vi "NanonisHelper_v1.vi"() -> ()   [LabVIEW 2014]
uses:
  <userlib>/Nanonis Prog Interface V5/Nanonis Prog Interface.lvlib
panel:
  in  "milliseconds to wait":u32=2
  in  "PLL":bool
  in  "size/pixel ratio":bool
  out "TCryo":dbl
  in  "Bias (V)":sgl min=-3.2 max=3.4 format="%#_5p"
  in  "set Bias":bool
  in  "Ratio":enum32{"Equal", "Independent"}(radio)
  out "Path":string="D:\\STM Data\\102016"
  in  "tilt from last image":bool
  out "millisecond timer value":u32=275798
  out "STM [K]":dbl=4.5364351144286035
  in  "polling msec":i32=3000
  in  "Speed (m/s)":cluster{"Forward":sgl, "Backward":sgl}={"Forward"=5.8593752e-08, "Backward"=5.8593752e-08} {"Backward" min=1e-15 max=3.5e-07 format="%.2p"; "Forward" min=1e-15 max=1.5e-07 format="%.2p"}
  in  "Prepare Topos":bool
  in  "Const Height":bool
  out "Saved file path":path=path "D:/STM Data/082016/160804_11-43-53_SPM001.sxm"
  out "Scanning":bool
  in  "up/down":bool=TRUE
  in  "Scan":bool
  in  "STS calc":bool
  in  "Tip cleaner":bool
  out "zdrift m/s":dbl format="%#_5p"
  in  "Duration":dbl
  in  "Z Drift":bool
  in  "stop":bool
  in  "Retract & Center":bool
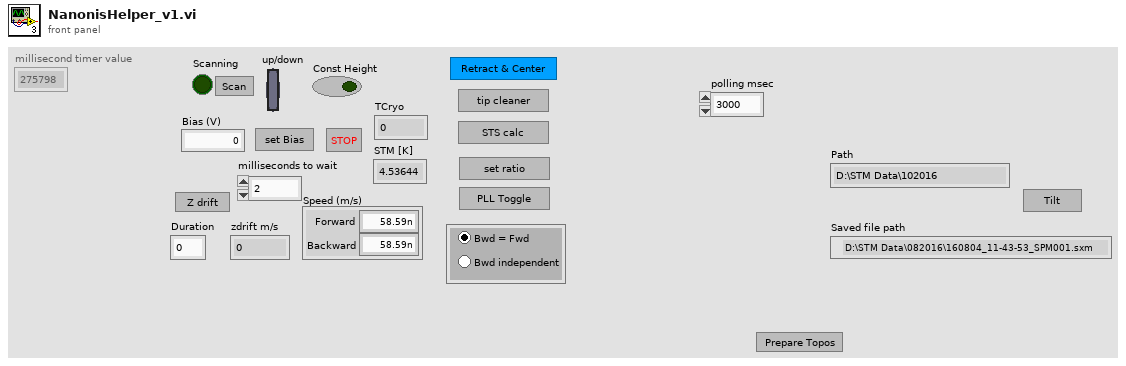
[diagram p1: front panel]
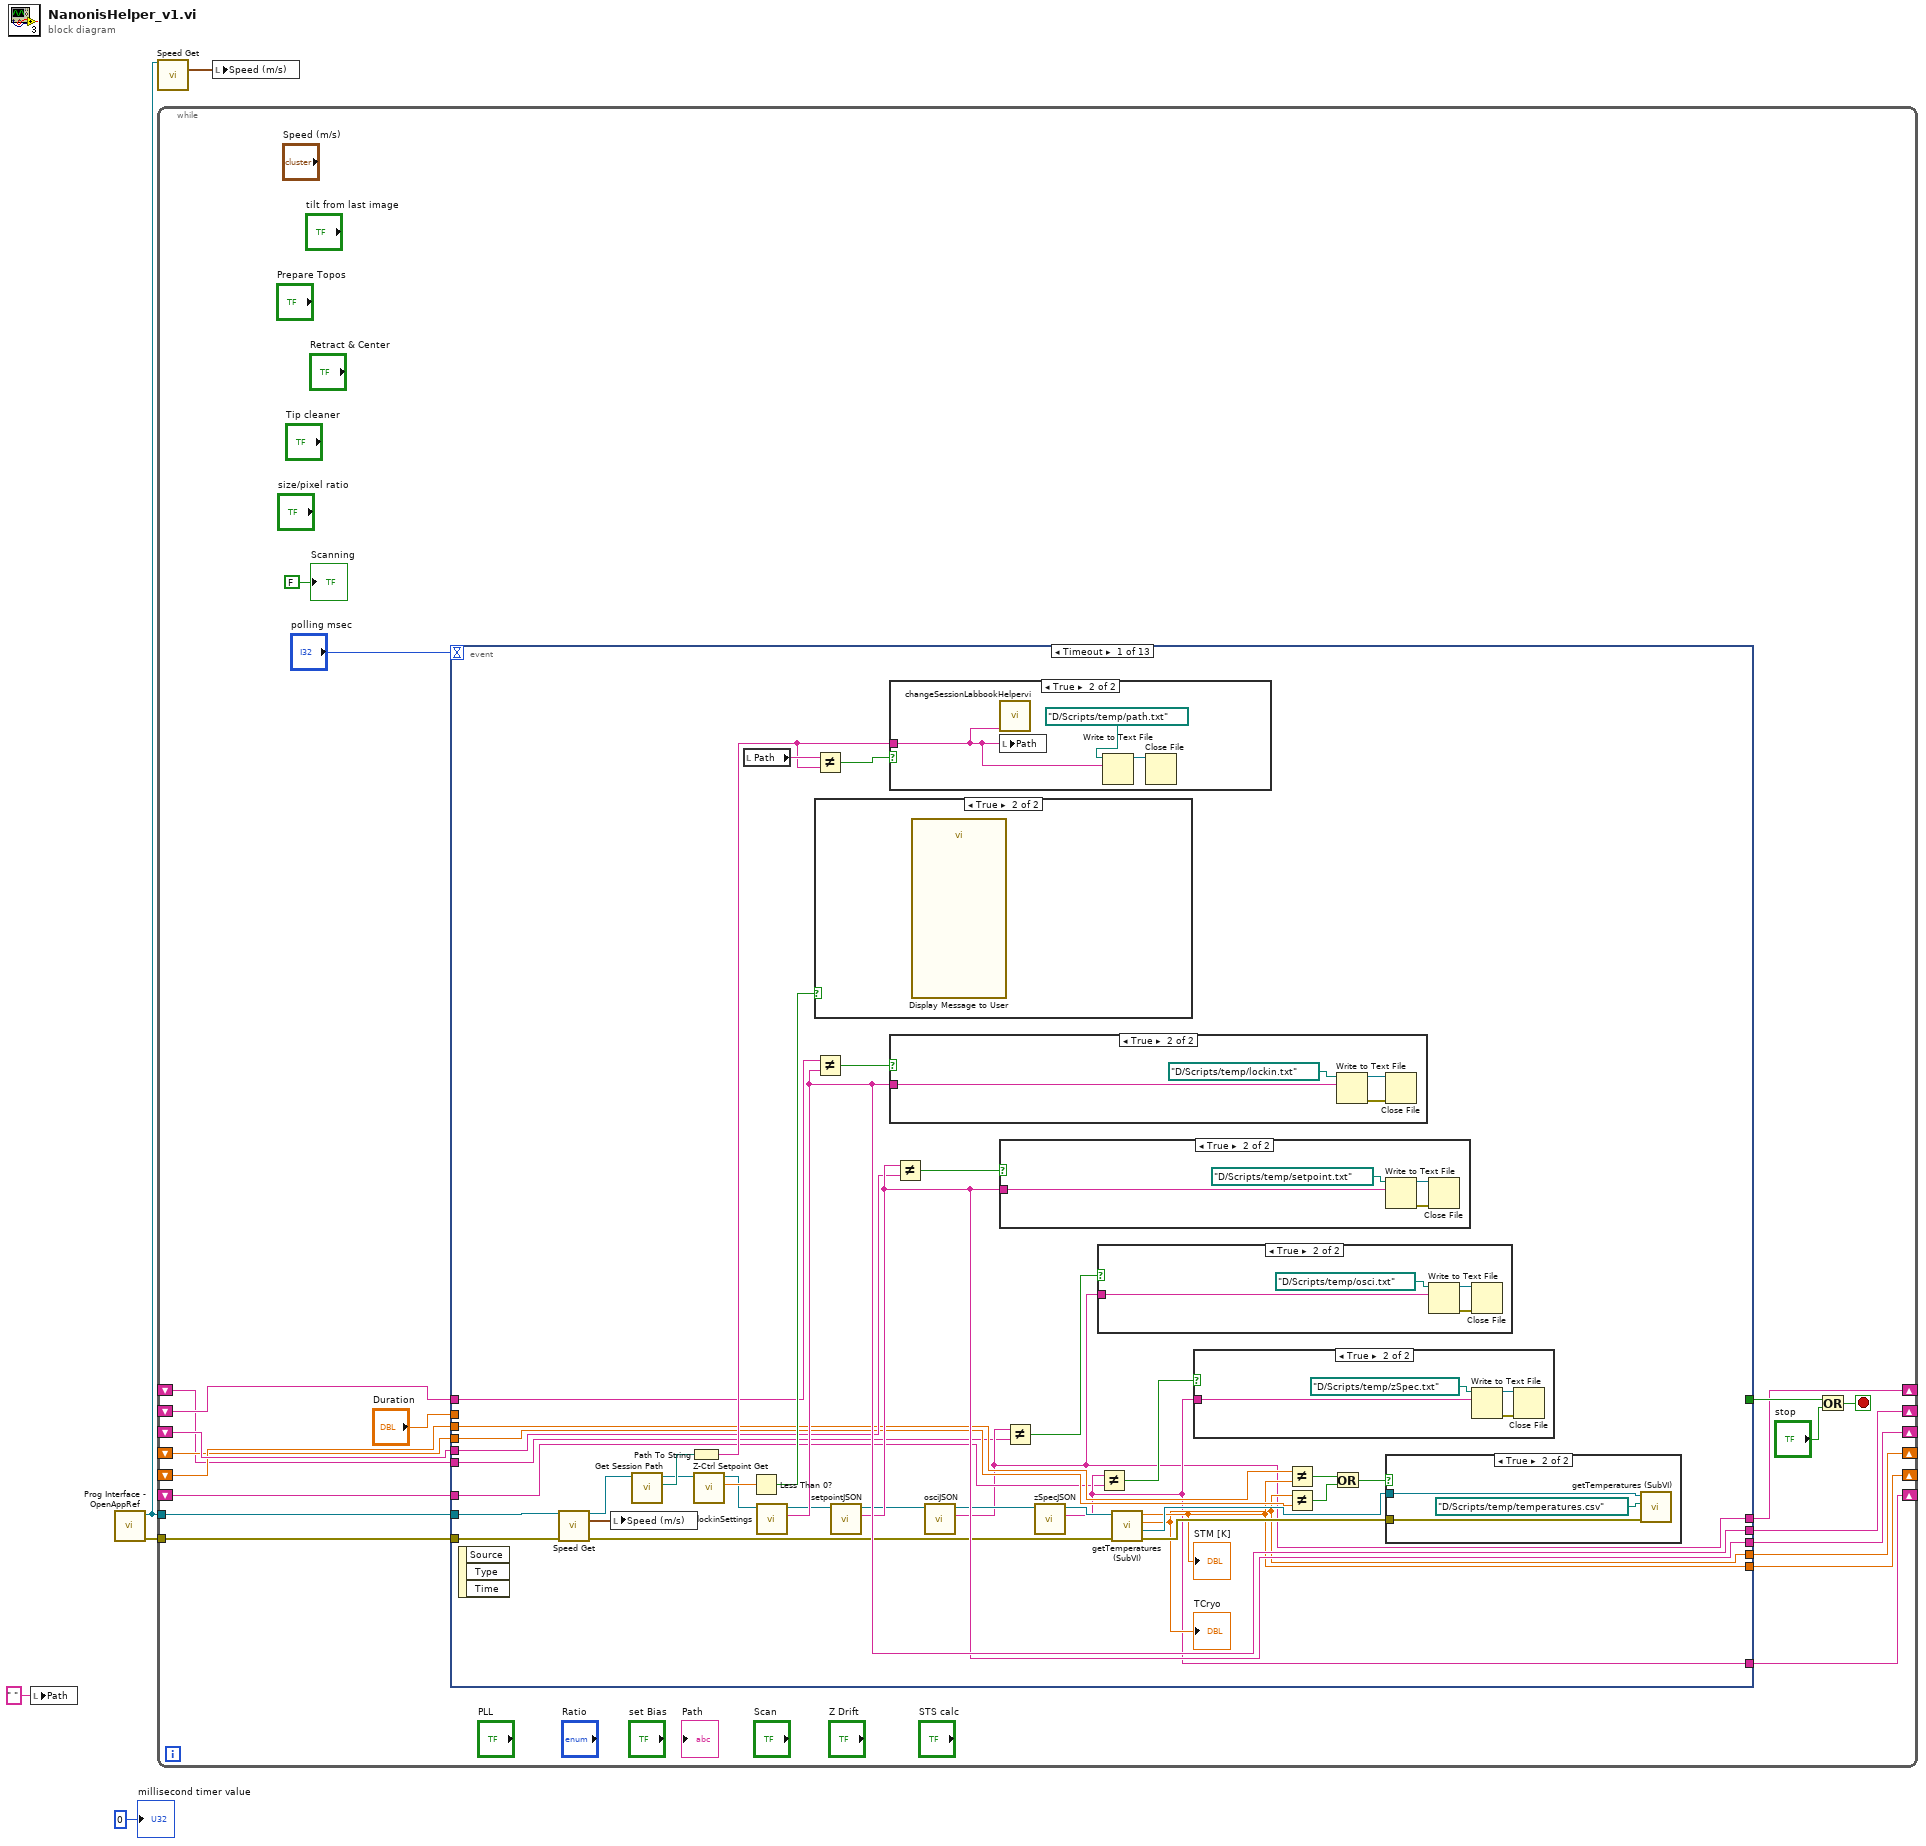
[diagram p0: block diagram]
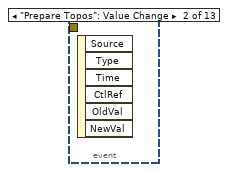
[diagram p9: hidden frame]
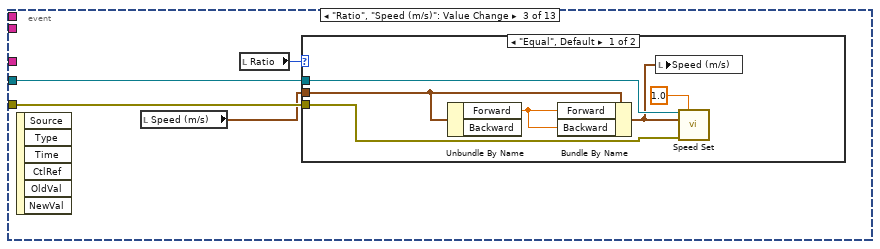
[diagram p10: hidden frame]
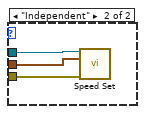
[diagram p11: hidden frame]
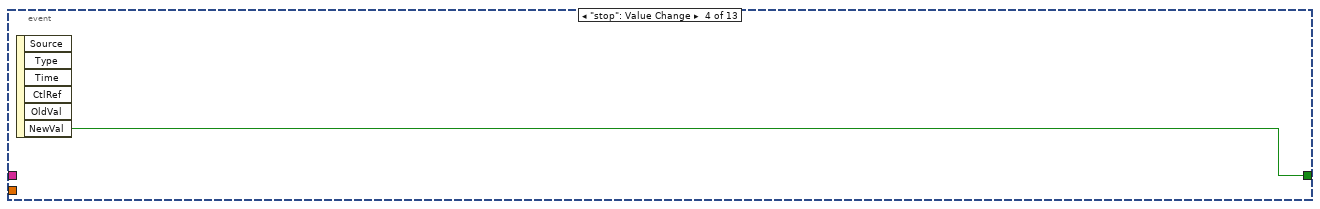
[diagram p12: hidden frame]
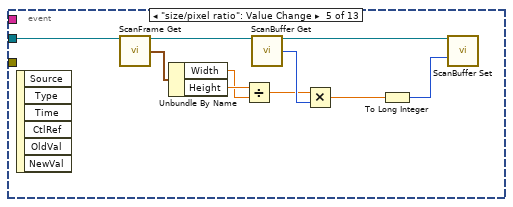
[diagram p13: hidden frame]
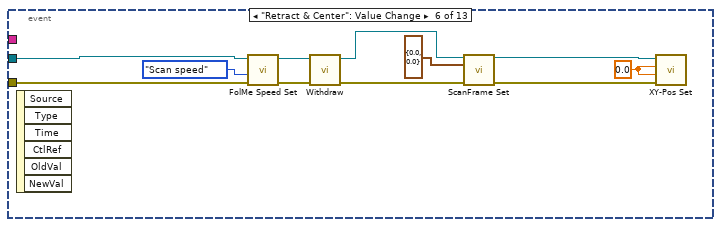
[diagram p14: hidden frame]
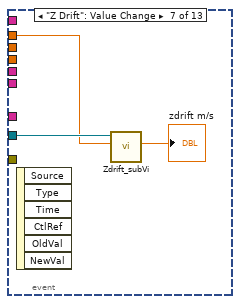
[diagram p15: hidden frame]
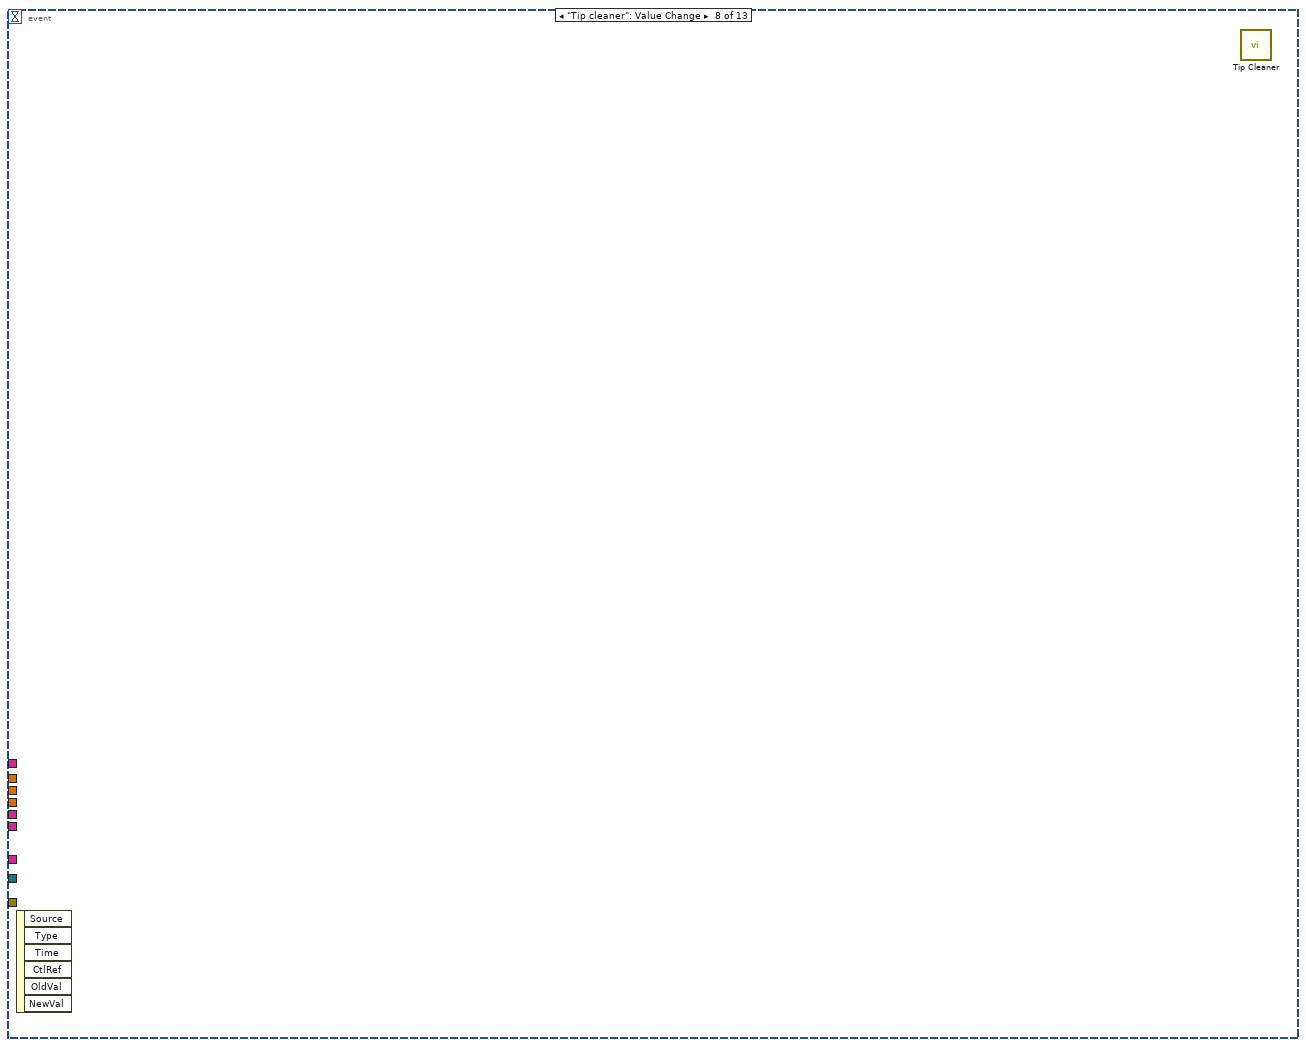
[diagram p16: hidden frame]
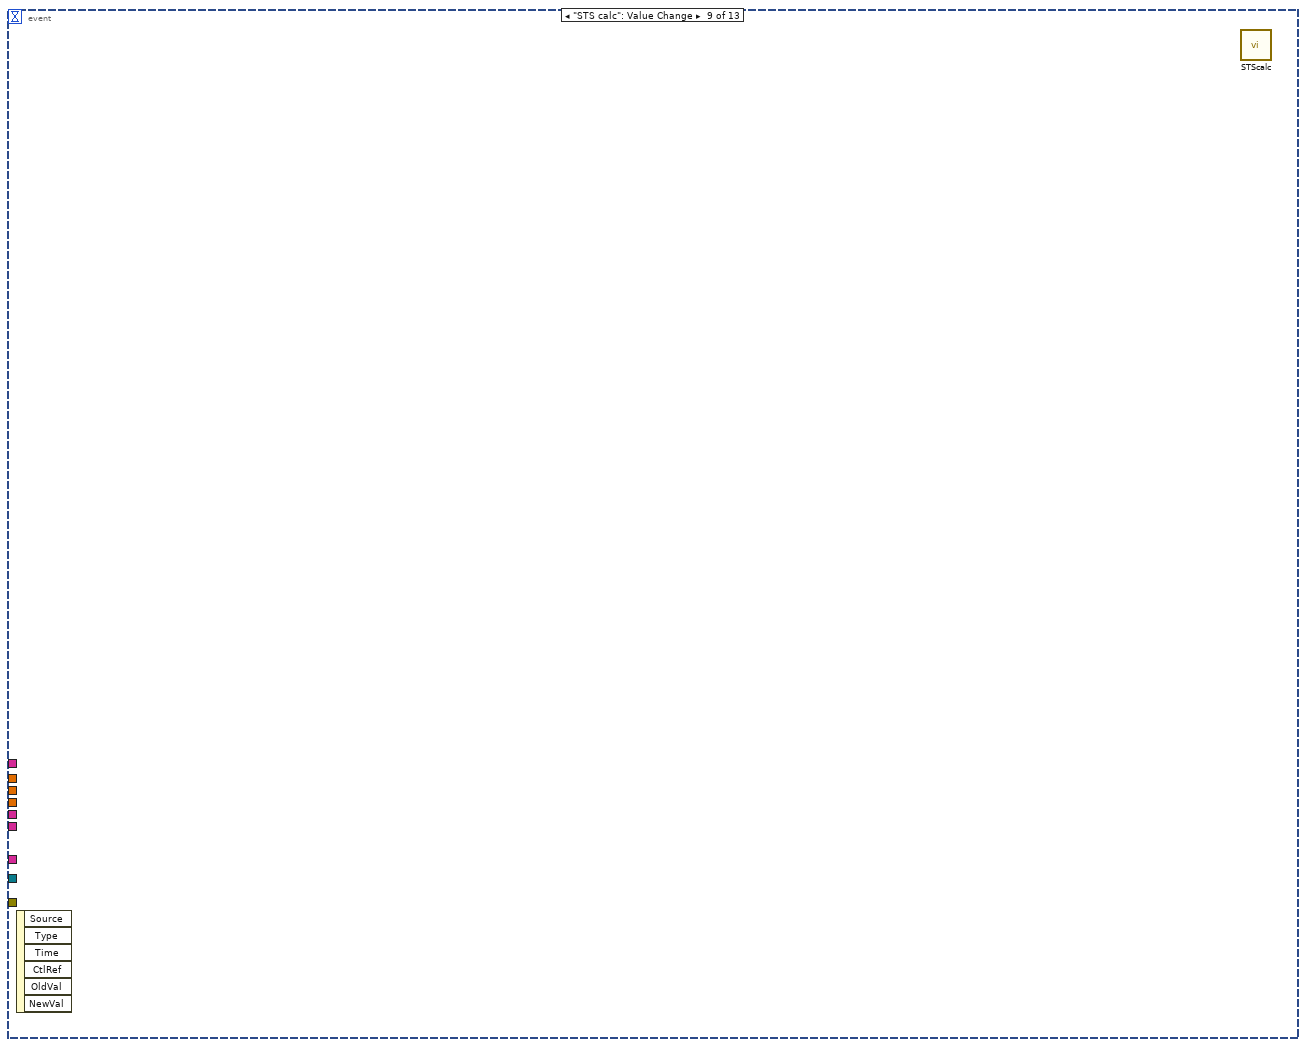
[diagram p17: hidden frame]
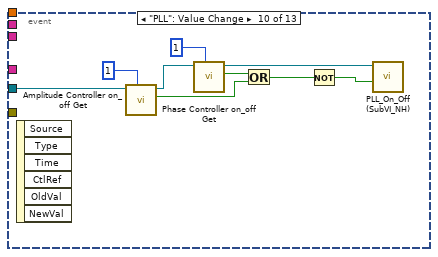
[diagram p18: hidden frame]
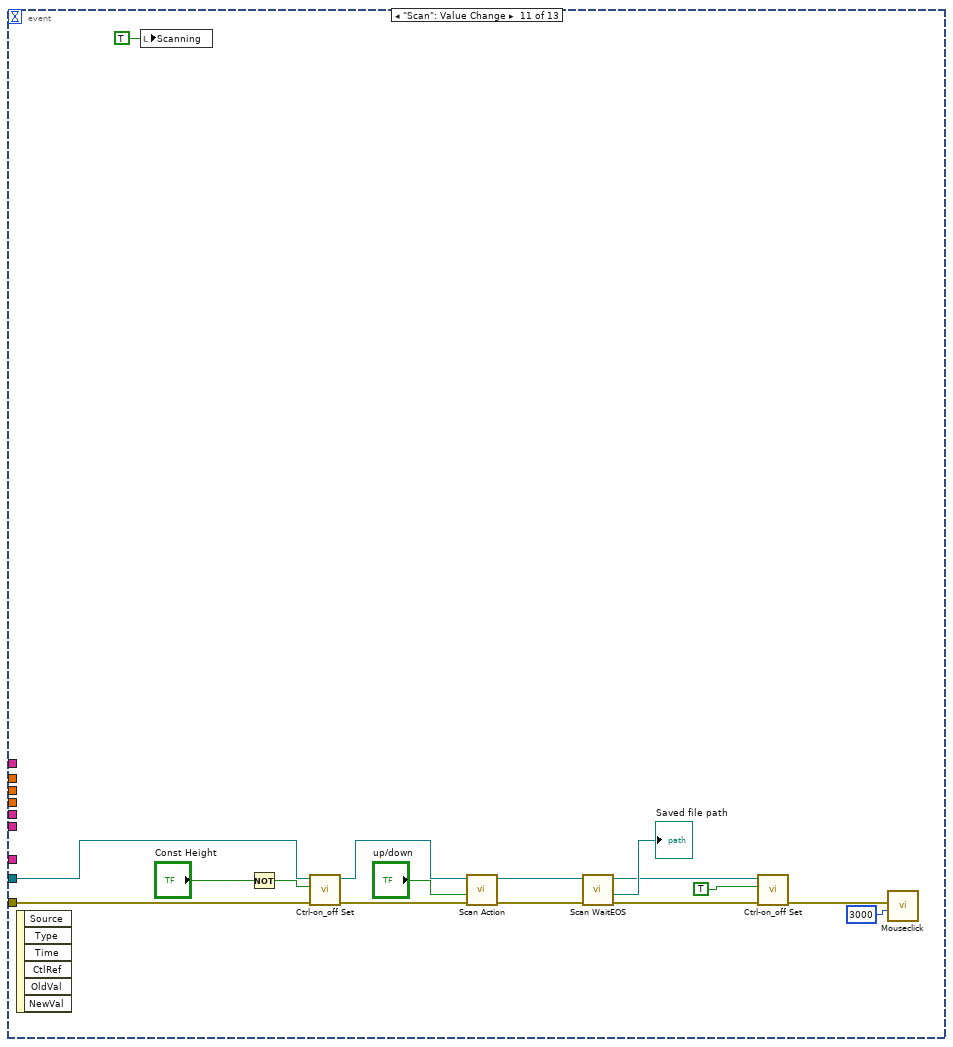
[diagram p19: hidden frame]
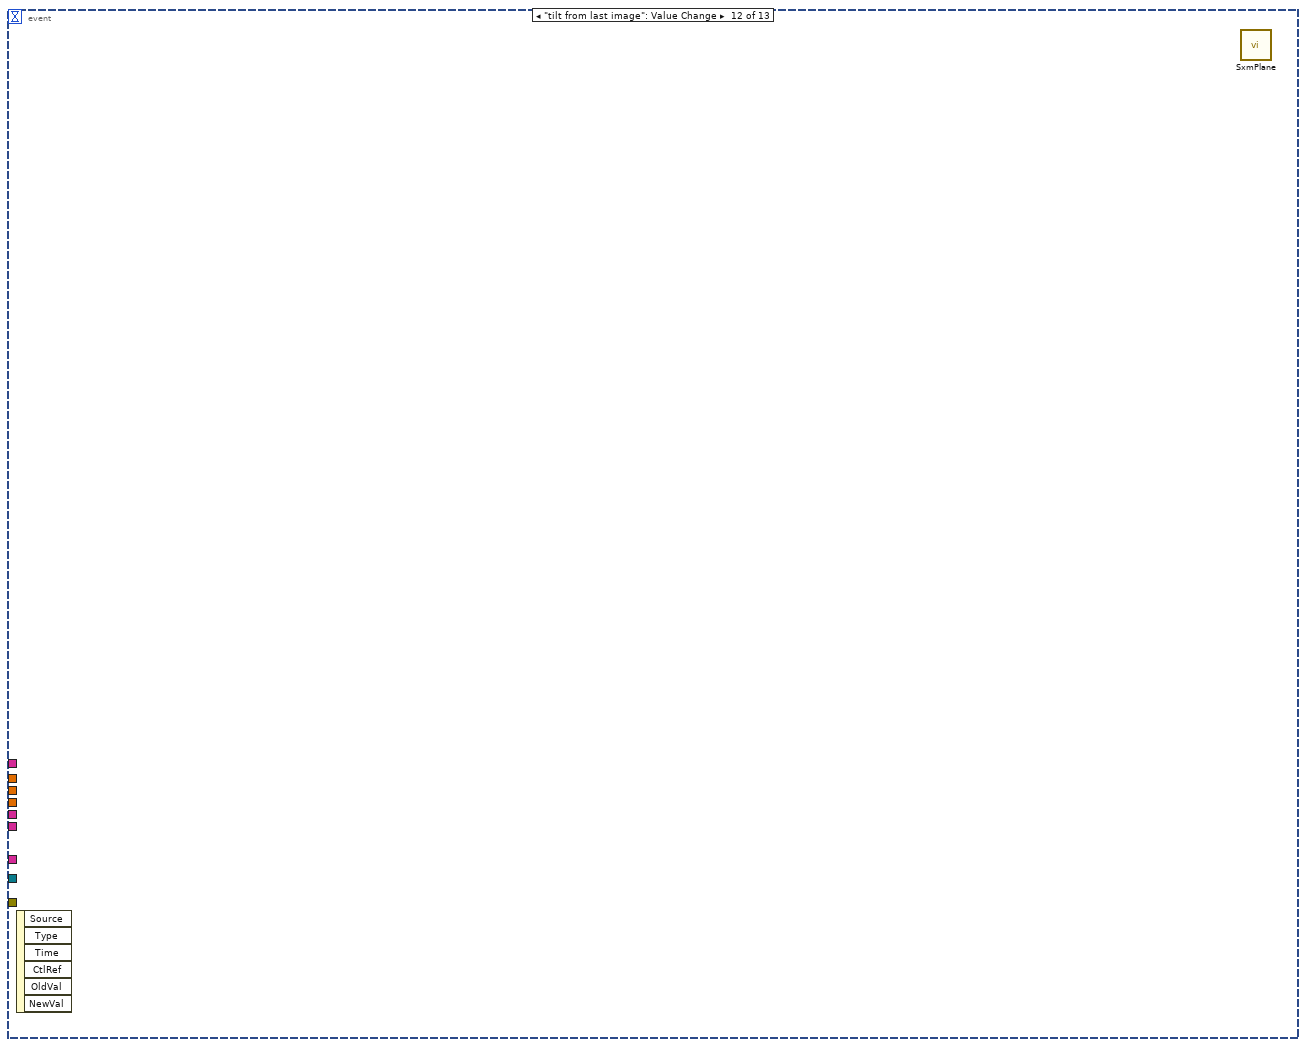
[diagram p20: hidden frame]
diagram:
  n1 = local write "Path"(" " ("Path")) -> ()
  n2 = call <userlib>:"Prog Interface - OpenAppRef.vi"() -> ("Error out"=w5:errorcluster, "Application reference"=w4:refnum<vi>)  [unwired: 6 in]
  n3 = call <userlib>:"Speed Get.vi"("Application ref in"=w4) -> ("Speed (m/s)"=w3:cluster{"Forward":sgl, "Backward":sgl})  [unwired: 9 in, 5 out]
  n4 = while {
    tunnel: w4 -> [w21]
    tunnel: w5 -> [w20]
    shift-right: [w17] -> _
    shift-left: _ -> [w16]
    shift-right: [w15] -> _
    shift-left: _ -> [w14]
    shift-right: [w13] -> _
    shift-left: _ -> [w12]
    shift-right: [w11] -> _
    shift-left: _ -> [w10]
    shift-right: [w8] -> _
    shift-left: _ -> [w7]
    shift-right: [w9] -> _
    shift-left: _ -> [w6]
    stop <- w19 stop-if-true
    n5 = event shown="[0] Timeout" {
      selector: _ -> [_ _ _ _ _ _ _ _ _ _ _ _ _]
      dyn-events: _ -> [_ _ _ _ _ _ _ _ _ _ _ _ _]
      timeout: "polling msec" -> [_ _ _ _ _ _ _ _ _ _ _ _ _]
      tunnel: w21 -> [w63 _ w89 _ w109 w113 w123 _ _ w132 w142 _ w152]
      tunnel: w20 -> [w62 _ w88 _ _ w111 _ _ _ _ w140 _ w149]
      tunnel: "Duration" -> [_ _ _ _ _ _ w121 _ _ _ _ _ _]
      tunnel: [_ _ _ w99 _ _ _ _ _ _ _ _ _] -> w24
      tunnel: [w52 _ _ _ _ _ _ _ _ _ _ _ _] -> w17
      tunnel: w16 -> [w53 _ _ _ _ _ _ _ _ _ _ _ _]
      tunnel: [w50 _ _ _ _ _ _ _ _ _ _ _ _] -> w15
      tunnel: w14 -> [w49 _ _ _ _ _ _ _ _ _ _ _ _]
      tunnel: [w40 _ _ _ _ _ _ _ _ _ _ _ _] -> w13
      tunnel: w12 -> [w47 _ _ _ _ _ _ _ _ _ _ _ _]
      tunnel: [w39 _ _ _ _ _ _ _ _ _ _ _ _] -> w11
      tunnel: w10 -> [w43 _ _ _ _ _ _ _ _ _ _ _ _]
      tunnel: [w28 _ _ _ _ _ _ _ _ _ _ _ _] -> w9
      tunnel: [w31 _ _ _ _ _ _ _ _ _ _ _ _] -> w8
      tunnel: w7 -> [w29 _ _ _ _ _ _ _ _ _ _ _ _]
      tunnel: w6 -> [w26 _ _ _ _ _ _ _ _ _ _ _ _]
      event Timeout {
        n6 = event-data() -> ()  [unwired: 1 in, 3 out]
        n7 = call <userlib>:"Speed Get.vi"("Application ref in"=w63, "error in (no error)"=w62) -> ("Application ref out"=w35:refnum<vi>, "Speed (m/s)"=w36:cluster{"Forward":sgl, "Backward":sgl}, "error out"=w45:errorcluster)  [unwired: 8 in, 3 out]
        n8 = local write "Speed (m/s)"(w36) -> ()
        n9 = call <userlib>:"Get Session Path.vi"("Application ref in"=w35) -> ("Session path"=w61:path, "Application ref out"=w55:refnum<vi>)  [unwired: 8 in, 1 out]
        n10 = Path To String(path=w61) -> (string=w58:string)
        n11 = call <userlib>:"Z-Ctrl Setpoint Get.vi"("Application ref in"=w55) -> ("Z Controller setpoint"=w56:sgl, "Application ref out"=w54:refnum<vi>)  [unwired: 7 in, 1 out]
        n12 = local read "Path"() -> (w60:string)
        n13 = Less Than 0?(x=w56) -> (x < 0?=w57:bool)
        n14 = call "lockinSettings.vi"("Application ref in"=w54) -> ("concatenated string"=w52:string, "Application ref out"=w37:refnum<vi>)  [unwired: 6 in, 1 out]
        n15 = Not Equal?(x=w60, y=w58) -> (x != y?=w59:bool)
        n16 = case shown="True" w57 {
          frame False {
          }
          frame True {
            n17 = call "Display Message to User"() -> ()  [unwired: 10 in, 2 out]
          }
        }
        n18 = Not Equal?(x=w53, y=w52) -> (x != y?=w51:bool)
        n19 = call "setpointJSON.vi"("Application ref in"=w37) -> ("JSON string"=w50:string, "Application ref out"=w34:refnum<vi>)  [unwired: 8 in, 1 out]
        n20 = case shown="True" w59 {
          tunnel: w58 -> [_ w85]
          frame False {
          }
          frame True {
            n21 = call "changeSessionLabbookHelpervi.vi"("strControlText"=w85) -> ()  [unwired: 10 in, 1 out]
            n22 = local write "Path"(w85) -> ()
            n23 = Write to Text File(file (use dialog)=path "D:/Scripts/temp/path.txt" ("file path (dialog if empty)"), text=w85) -> (refnum out=w83:refnum<file>)  [unwired: 2 in, 2 out]
            n24 = Close File(refnum=w83) -> ()  [unwired: 1 in, 2 out]
          }
        }
        n25 = case shown="True" w51 {
          tunnel: w52 -> [_ w79]
          frame False {
          }
          frame True {
            n26 = Write to Text File(file (use dialog)=path "D:/Scripts/temp/lockin.txt" ("file path (dialog if empty)"), text=w79) -> (refnum out=w80:refnum<file>, error out=w81:errorcluster)  [unwired: 2 in, 1 out]
            n27 = Close File(refnum=w80, error in=w81) -> ()  [unwired: 2 out]
          }
        }
        n28 = Not Equal?(x=w50, y=w49) -> (x != y?=w48:bool)
        n29 = call "osciJSON.vi"("Application ref in"=w34) -> ("JSON string"=w28:string, "Application ref out"=w33:refnum<vi>)  [unwired: 8 in, 1 out]
        n30 = case shown="True" w48 {
          tunnel: w50 -> [_ w75]
          frame False {
          }
          frame True {
            n31 = Write to Text File(file (use dialog)=path "D:/Scripts/temp/setpoint.txt" ("file path (dialog if empty)"), text=w75) -> (refnum out=w76:refnum<file>, error out=w78:errorcluster)  [unwired: 2 in, 1 out]
            n32 = Close File(refnum=w76, error in=w78) -> ()  [unwired: 2 out]
          }
        }
        n33 = Not Equal?(x=w28, y=w26) -> (x != y?=w27:bool)
        n34 = call "zSpecJSON.vi"("Application ref in"=w33) -> ("JSON string"=w31:string, "Application ref out"=w32:refnum<vi>)  [unwired: 8 in, 1 out]
        n35 = case shown="True" w27 {
          tunnel: w28 -> [_ w64]
          frame False {
          }
          frame True {
            n36 = Write to Text File(file (use dialog)=path "D:/Scripts/temp/osci.txt" ("file path (dialog if empty)"), text=w64) -> (refnum out=w65:refnum<file>, error out=w67:errorcluster)  [unwired: 2 in, 1 out]
            n37 = Close File(refnum=w65, error in=w67) -> ()  [unwired: 2 out]
          }
        }
        n38 = Not Equal?(x=w31, y=w29) -> (x != y?=w30:bool)
        n39 = call "getTemperatures (SubVI).vi"("error in (no error)"=w45, "Application in"=w32) -> ("error out"=w44:errorcluster, "Application ref out"=w46:refnum<vi>, "TCryo"=w39:dbl, "TSTM"=w40:dbl)  [unwired: 6 in]
        "STM [K]" <- w40
        "TCryo" <- w39
        n40 = case shown="True" w30 {
          tunnel: w31 -> [_ w68]
          frame False {
          }
          frame True {
            n41 = Write to Text File(file (use dialog)=path "D:/Scripts/temp/zSpec.txt" ("file path (dialog if empty)"), text=w68) -> (refnum out=w69:refnum<file>, error out=w71:errorcluster)  [unwired: 2 in, 1 out]
            n42 = Close File(refnum=w69, error in=w71) -> ()  [unwired: 2 out]
          }
        }
        n43 = Not Equal?(x=w47, y=w40) -> (x != y?=w42:bool)
        n44 = Not Equal?(x=w39, y=w43) -> (x != y?=w41:bool)
        n45 = Or(x=w42, y=w41) -> (x .or. y?=w38:bool)
        n46 = case shown="True" w38 {
          tunnel: w46 -> [_ w73]
          tunnel: w44 -> [_ w72]
          frame False {
          }
          frame True {
            n47 = call "getTemperatures (SubVI).vi"("error in (no error)"=w72, "file path (dialog if empty)"=path "D:/Scripts/temp/temperatures.csv", "Application in"=w73) -> ()  [unwired: 5 in, 4 out]
          }
        }
      }
      event "Prepare Topos": Value Change {
        n48 = event-data() -> ()  [unwired: 1 in, 6 out]
      }
      event "Ratio", "Speed (m/s)": Value Change {
        n49 = event-data() -> ()  [unwired: 1 in, 6 out]
        n50 = local read "Speed (m/s)"() -> (w87:cluster{"Forward":sgl, "Backward":sgl})
        n51 = local read "Ratio"() -> (w86:enum32{"Equal", "Independent"})
        n52 = case shown="\"Equal\", Default" w86 {
          tunnel: w87 -> [w94 w98]
          tunnel: w89 -> [w92 w97]
          tunnel: w88 -> [w95 w96]
          frame "Equal", Default {
            n53 = Unbundle By Name(w94) -> ("Forward"=w93:sgl)  [unwired: 1 out]
            n54 = Bundle By Name(cluster=w94, "Forward"=w93, "Backward"=w93) -> (w91:cluster{"Forward":sgl, "Backward":sgl})
            n55 = local write "Speed (m/s)"(w91) -> ()
            n56 = call <userlib>:"Speed Set.vi"("Application ref in"=w92, "Speed ratio"=sgl 1.0, "Speed (m/s)"=w91, "error in (no error)"=w95) -> ()  [unwired: 10 in, 2 out]
          }
          frame "Independent" {
            n57 = call <userlib>:"Speed Set.vi"("Application ref in"=w97, "Speed (m/s)"=w98, "error in (no error)"=w96) -> ()  [unwired: 11 in, 2 out]
          }
        }
      }
      event "stop": Value Change {
        n58 = event-data() -> ("NewVal"=w99:bool)  [unwired: 1 in, 5 out]
      }
      event "size/pixel ratio": Value Change {
        n59 = event-data() -> ()  [unwired: 1 in, 6 out]
        n60 = call <userlib>:"ScanFrame Get.vi"("Application ref in"=w109) -> ("Application ref out"=w107:refnum<vi>, "Size (m)"=w108:cluster{"Width":sgl, "Height":sgl})  [unwired: 10 in, 3 out]
        n61 = Unbundle By Name(w108) -> ("Width"=w101:sgl, "Height"=w102:sgl)
        n62 = Divide(x=w102, y=w101) -> (x/y=w103:sgl)
        n63 = call <userlib>:"ScanBuffer Get.vi"("Application ref in"=w107) -> ("Application ref out"=w106:refnum<vi>, "Pixels/line"=w105:i32)  [unwired: 10 in, 3 out]
        n64 = Multiply(x=w103, y=w105) -> (x*y=w104:sgl)
        n65 = To Long Integer(number=w104) -> (32bit integer=w100:i32)
        n66 = call <userlib>:"ScanBuffer Set.vi"("Application ref in"=w106, "Lines"=w100) -> ()  [unwired: 12 in, 2 out]
      }
      event "Retract & Center": Value Change {
        w115 = sgl 0.0 ("X (m)")
        n67 = event-data() -> ()  [unwired: 1 in, 6 out]
        n68 = call <userlib>:"FolMe Speed Set.vi"("error in (no error)"=w111, "Speed Setting (Custom)"=enum32{"Scan speed", "Custom speed"}."Scan speed", "Application ref in"=w113) -> ("error out"=w110:errorcluster, "Application ref out"=w112:refnum<vi>)  [unwired: 5 in]
        n69 = call <userlib>:"Withdraw.vi"("Error in (no error)"=w110, "Application ref in"=w112) -> ("Error out"=w119:errorcluster, "Application ref out"=w120:refnum<vi>)  [unwired: 8 in]
        n70 = call <userlib>:"ScanFrame Set.vi"("Application ref in"=w120, "Center coordinates (m)"=cluster{"Xc":sgl, "Yc":sgl} {"Xc"=0.0, "Yc"=0.0}, "error in (no error)"=w119) -> ("Application ref out"=w116:refnum<vi>, "error out"=w117:errorcluster)  [unwired: 11 in]
        n71 = call <userlib>:"XY-Pos Set.vi"("error in (no error)"=w117, "Y (m)"=w115, "X (m)"=w115, "Application ref in"=w116) -> ()  [unwired: 4 in, 2 out]
      }
      event "Z Drift": Value Change {
        n72 = event-data() -> ()  [unwired: 1 in, 6 out]
        n73 = call "Zdrift_subVi.vi"("Duration"=w121, "Application in"=w123) -> ("z drift"=→"zdrift m/s":dbl)  [unwired: 7 in, 2 out]
      }
      event "Tip cleaner": Value Change {
        n74 = event-data() -> ()  [unwired: 1 in, 6 out]
        n75 = call <userlib>:"Tip Cleaner.vi"() -> ()  [unwired: 1 in]
      }
      event "STS calc": Value Change {
        n76 = event-data() -> ()  [unwired: 1 in, 6 out]
        n77 = call "STScalc.vi"() -> ()  [unwired: 12 in]
      }
      event "PLL": Value Change {
        n78 = event-data() -> ()  [unwired: 1 in, 6 out]
        n79 = call <userlib>:"Amplitude Controller on_off Get.vi"("Modulator index"=1, "Application ref in"=w132) -> ("Amplitude controller on/off status"=w128:bool, "Application ref out"=w131:refnum<vi>)  [unwired: 7 in, 1 out]
        n80 = call <userlib>:"Phase Controller on_off Get.vi"("Modulator index"=1, "Application ref in"=w131) -> ("Phase controller on/off status"=w127:bool, "Application ref out"=w125:refnum<vi>)  [unwired: 7 in, 1 out]
        n81 = Or(x=w127, y=w128) -> (x .or. y?=w126:bool)
        n82 = Not(x=w126) -> (.not. x?=w124:bool)
        n83 = call "PLL_On_Off (SubVI_NH).vi"("Output ON/OFF (F=OFF)"=w124, "Application in"=w125) -> ()  [unwired: 8 in, 2 out]
      }
      event "Scan": Value Change {
        n84 = event-data() -> ()  [unwired: 1 in, 6 out]
        n85 = local write "Scanning"(TRUE ("Scanning")) -> ()
        n86 = Not(x="Const Height") -> (.not. x?=w134:bool)
        n87 = call <userlib>:"Ctrl-on_off Set.vi"("error in (no error)"=w140, "Z Controller ON/OFF"=w134, "Application ref in"=w142) -> ("error out"=w139:errorcluster, "Application ref out"=w141:refnum<vi>)  [unwired: 7 in]
        n88 = call <userlib>:"Scan Action.vi"("error in (no error)"=w139, "Direction: up/down (T=up)"="up/down", "Application ref in"=w141) -> ("error out"=w147:errorcluster, "Application ref out"=w146:refnum<vi>)  [unwired: 6 in]
        n89 = call <userlib>:"Scan WaitEOS.vi"("error in (no error)"=w147, "Application ref in"=w146) -> ("error out"=w136:errorcluster, "Saved file path"=→"Saved file path":path, "Application ref out"=w138:refnum<vi>)  [unwired: 5 in, 1 out]
        n90 = call <userlib>:"Ctrl-on_off Set.vi"("error in (no error)"=w136, "Z Controller ON/OFF"=TRUE, "Application ref in"=w138) -> ("error out"=w137:errorcluster)  [unwired: 7 in, 1 out]
        n91 = call "Mouseclick.vi"("nMilliseconds"=3000, "error in (no error)"=w137) -> ()  [unwired: 9 in, 1 out]
      }
      event "tilt from last image": Value Change {
        n92 = event-data() -> ()  [unwired: 1 in, 6 out]
        n93 = call "SxmPlane.vi"() -> ()  [unwired: 12 in]
      }
      event "set Bias": Value Change {
        n94 = event-data() -> ()  [unwired: 1 in, 6 out]
        n95 = Not Equal To 0?(x="Bias (V)") -> (x != 0?=w150:bool)
        n96 = case shown="True" w150 {
          tunnel: w152 -> [_ w156]
          tunnel: "Bias (V)" -> [_ w155]
          tunnel: w149 -> [_ w154]
          frame False {
          }
          frame True {
            n97 = call "SafeBiasSet.vi"("Application ref in"=w156, "Bias (V)"=w155, "error in (no error)"=w154, "milliseconds to wait"="milliseconds to wait") -> ()  [unwired: 5 in, 2 out]
          }
        }
      }
    }
    n98 = Or(x=w24, y="stop") -> (x .or. y?=w19:bool)
    "Scanning" <- FALSE ("Scanning")
  }
  n99 = local write "Speed (m/s)"(w3) -> ()
  "millisecond timer value" <- u32 0 ("millisecond timer value")
